vi "create_full_request_data.vi"(0 "llm_openai_chatmodels in":refnum<class "llm_openai_chatmodels.lvclass">, 5 "Messages":refnum<class "abstract_message_base.lvclass">[](array[class]), 11 "error in (no error)":errorcluster) -> (4 "llm_openai_chatmodels out":refnum<class "llm_openai_chatmodels.lvclass">, 6 "Request Data":string, 15 "error out":errorcluster)   [LabVIEW 2020, in "llm_openai_chatmodels.lvclass"]
uses:
  llm_openai_chatmodels.lvclass
  D:/Personal/LabVIEW LLMs/src/models/abstract_llm_base/abstract_llm_base.lvclass
  abstract_message_base/abstract_message_base.lvclass
  utils/openai_chatmodel_request_data.ctl
  llm_openai_chatmodels.lvclass/llm_openai_chatmodels.ctl
  message_text/message_text.lvclass
  message_image/message_image.lvclass
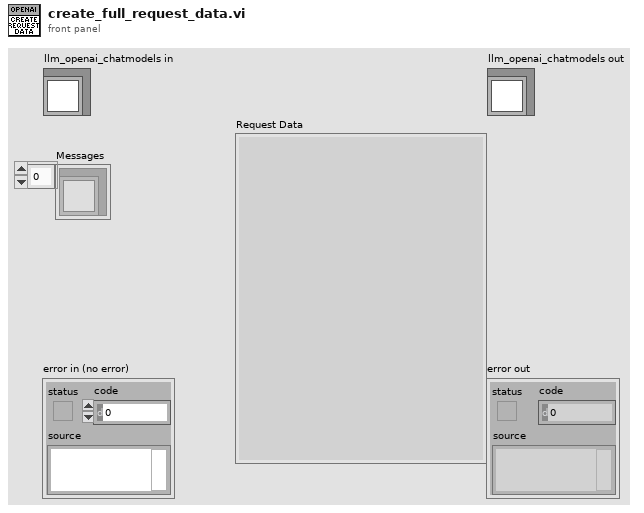
[diagram p1: front panel]
types:
  T1 = typedef "llm_openai_chatmodels.lvclass/openai_chatmodel_request_data.ctl" = cluster{"model":string, "messages":string, "temperature":dbl, "max_completion_tokens":u32, "top_p":dbl, "frequency_penalty":dbl, "presence_penalty":dbl, "response_format":cluster{"type":string}}
  T2 = typedef "message_text.lvclass/message.ctl" = cluster{"role":string, "content":string[]}
  T3 = cluster{"role":string, "content":cluster{"type":string, "text":string}[]}
  T4 = typedef "message_image.lvclass/message.ctl" = cluster{"role":string, "content_text":string[], "content_images":path[]}
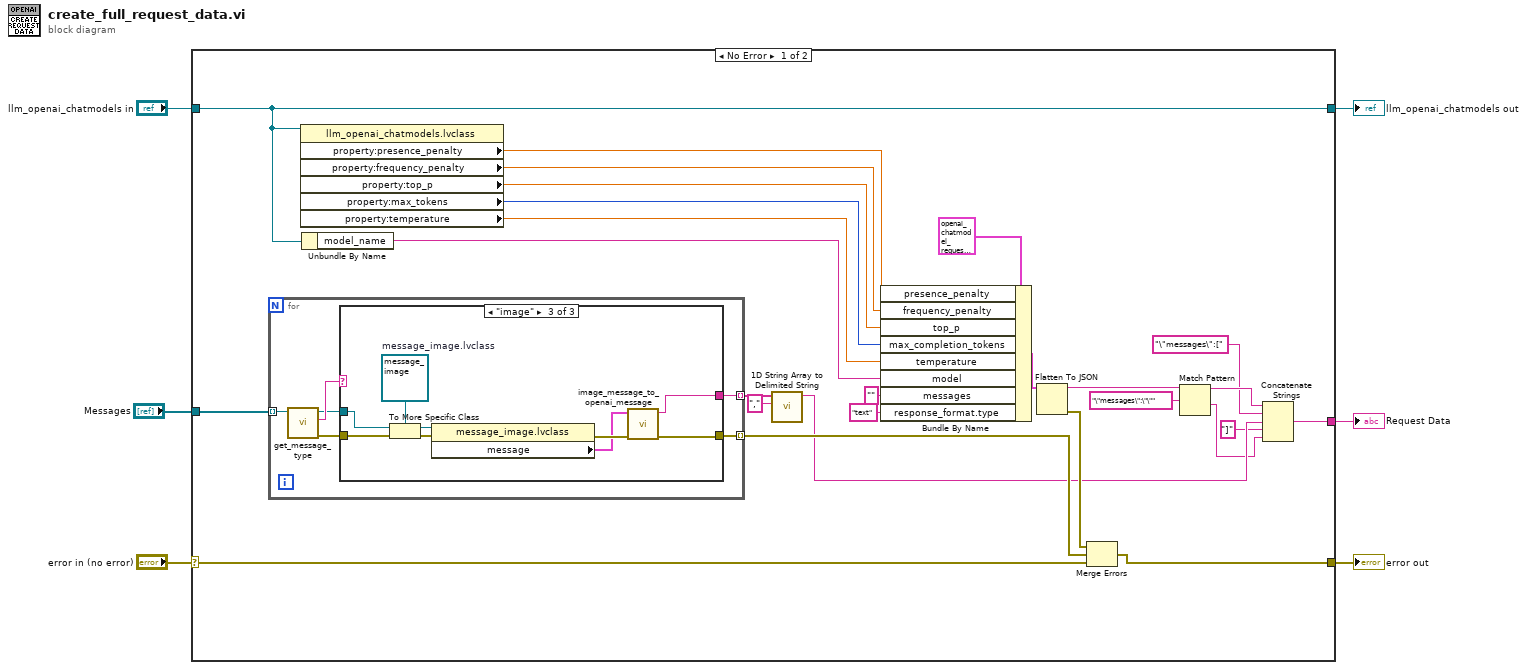
[diagram p0: block diagram]
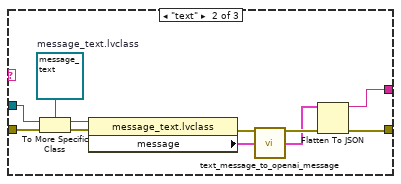
[diagram p3: hidden frame]
diagram:
  n1 = case shown="No Error" "error in (no error)" {
    selector: "error in (no error)" -> [w32 w60]
    tunnel: [w27 w60] -> w5
    tunnel: [w24 w59] -> w3
    tunnel: "llm_openai_chatmodels in" -> [w24 w59]
    tunnel: "Messages" -> [w29 _]
    tunnel: [w7 _] -> w1
    frame No Error {
      n2 = for {
        tunnel: w29 -> [w38] mode=indexing
        tunnel: [w34] -> w26 mode=indexing
        tunnel: [w33] -> w16 mode=indexing
        n3 = call-dynamic "get_message_type.vi"("abstract_message_base in"=w38) -> ("error out"=w35:errorcluster, "Type"=w37:string, "abstract_message_base out"=w36:refnum<class "abstract_message_base.lvclass">)  [unwired: 8 in]
        n4 = case shown="\"image\"" w37 {
          tunnel: w36 -> [_ w48 w54]
          tunnel: w35 -> [w39 w49 w55]
          tunnel: [w39 w42 w52] -> w34
          tunnel: [_ w40 w50] -> w33
          frame Default {
          }
          frame "text" {
            w47 = refnum<class "message_text.lvclass"> refnum  # message_text.lvclass
            n5 = To More Specific Class(target class=w47, reference=w48, error in=w49) -> (specific class reference=w46:refnum<class "message_text.lvclass">, error out=w45:errorcluster)
            n6 = property class="message_text.lvclass"(reference=w46, error in=w45) -> (error out=w43:errorcluster, "message"=w44:T2)  [unwired: 1 out]
            n7 = call "text_message_to_openai_message.vi"("message"=w44) -> ("message out"=w41:T3)
            n8 = Flatten To JSON(anything=w41, error in (no error)=w43) -> (JSON string=w40:string, 11:w42:errorcluster)  [unwired: 1 in]
          }
          frame "image" {
            w56 = refnum<class "message_image.lvclass"> refnum  # message_image.lvclass
            n9 = To More Specific Class(target class=w56, reference=w54, error in=w55) -> (specific class reference=w58:refnum<class "message_image.lvclass">, error out=w57:errorcluster)
            n10 = property class="message_image.lvclass"(reference=w58, error in=w57) -> (error out=w53:errorcluster, "message"=w51:T4)  [unwired: 1 out]
            n11 = call "image_message_to_openai_message.vi"("error in (no error)"=w53, "message"=w51) -> ("error out"=w52:errorcluster, "OpenAI message"=w50:string)  [unwired: 8 in]
          }
        }
      }
      n12 = property class="llm_openai_chatmodels.lvclass"(reference=w24) -> ("property:presence_penalty"=w22:dbl, "property:frequency_penalty"=w21:dbl, "property:top_p"=w20:dbl, "property:max_tokens"=w19:u32, "property:temperature"=w18:dbl)  [unwired: 1 in, 2 out]
      n13 = Unbundle By Name(w24) -> ("model_name"=w30:string)
      n14 = call <vilib>:"1D String Array to Delimited String.vi"("delimiter"=",", "string array"=w16) -> ("delimited string"=w10:string)  [unwired: 9 in]
      n15 = Bundle By Name(cluster=T1 {"model"="", "messages"="", "temperature"=1.0, "max_completion_tokens"=256, "top_p"=1.0, "frequency_penalty"=0.0, "presence_penalty"=0.0, "response_format"={"type"="text"}} ("data"), "presence_penalty"=w22, "frequency_penalty"=w21, "top_p"=w20, "max_completion_tokens"=w19, "temperature"=w18, "model"=w30, "messages"="", "response_format.type"="text") -> (w28:T1)
      n16 = Flatten To JSON(anything=w28) -> (JSON string=w12:string, 11:w25:errorcluster)  [unwired: 2 in]
      n17 = Merge Errors(w25, w26, w32) -> (w27:errorcluster)
      n18 = Match Pattern(string=w12, regular expression="\"messages\":\"\"") -> (before substring=w14:string, after substring=w8:string)  [unwired: 1 in, 2 out]
      n19 = Concatenate Strings(w14, "\"messages\":[", w10, "]" ("string"), w8) -> (w7:string)
    }
    frame Error {
    }
  }
  "error out" <- w5
  "llm_openai_chatmodels out" <- w3
  "Request Data" <- w1
